vi "Set Tree Items.vi"(8 "error in (no error)":errorcluster, 11 "File Explorer in":refnum<class "File Explorer.lvclass">) -> (0 "error out":errorcluster, 3 "File Explorer out":refnum<class "File Explorer.lvclass">)   [LabVIEW 2019, in "File Explorer.lvlib" / "File Explorer.lvclass"]
uses:
  <vilib>/gpm_packages/@cs/file-explorer-extension/Source/File Explorer/File Explorer/File Explorer.lvclass
  <vilib>/gpm_packages/@cs/file-explorer-extension/Source/File Explorer/File Explorer/File Explorer.lvclass/File Explorer.ctl
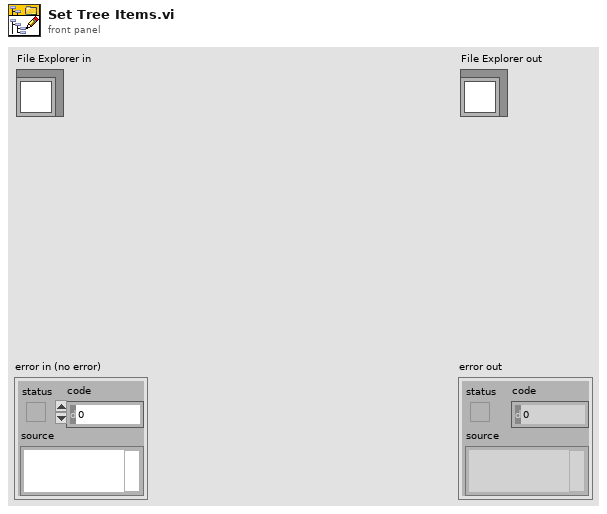
[diagram p1: front panel]
types:
  T1 = cluster{"Left Cell String":string, "Child Text":string[], "Child Tag":string, "Item Indent":i32, "Child Only?":bool, "Glyph Index":i32}[]
  T2 = cluster{"Left Cell String":string, "Child Text":string[], "Child Tag":string, "Item Indent":i32, "Child Only?":bool, "Glyph Index":i32}
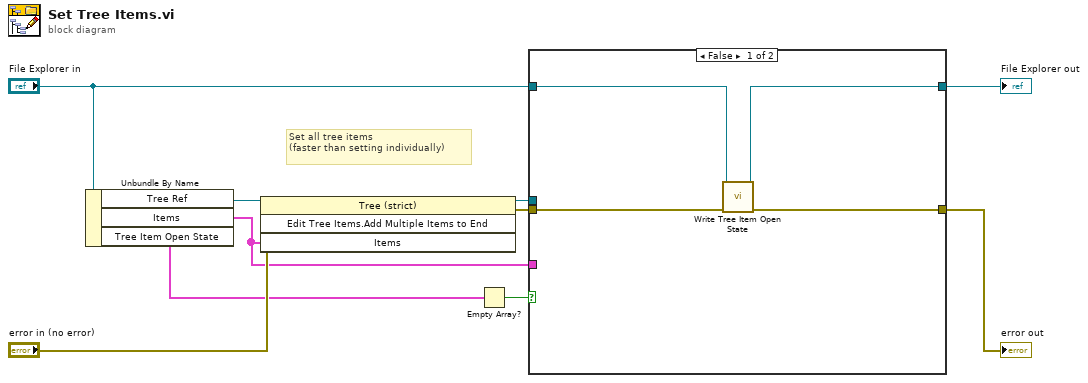
[diagram p0: block diagram]
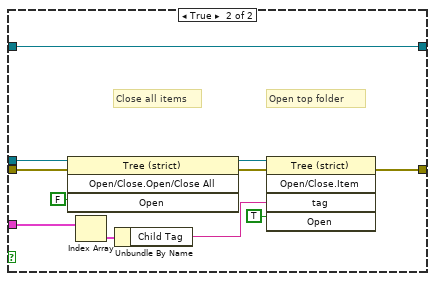
[diagram p2: hidden frame]
diagram:
  # "Set all tree items\n(faster than setting individually)"
  n1 = Unbundle By Name("File Explorer in") -> ("Tree Ref"=w6:refnum<vi>, "Items"=w5:T1, "Tree Item Open State"=w4:cluster{"Tag":string, "Open?":bool}[])
  n2 = invoke class="Tree (strict)" method="Edit Tree Items.Add Multiple Items to End"(reference=w6, error in="error in (no error)", "Items"=w5) -> (reference out=w9:refnum<vi>, error out=w10:errorcluster)  [unwired: 1 in, 2 out]
  n3 = Empty Array?(array=w4) -> (empty?=w3:bool)
  n4 = case shown="False" w3 {
    tunnel: w10 -> [w14 w25]
    tunnel: w9 -> [_ w24]
    tunnel: [w13 w17] -> w7
    tunnel: w5 -> [_ w16]
    tunnel: [w11 w15] -> w1
    tunnel: "File Explorer in" -> [w12 w15]
    frame False {
      n5 = call <vilib>:"Write Tree Item Open State.vi"("error in (no error)"=w14, "File Explorer in"=w12) -> ("error out"=w13:errorcluster, "File Explorer out"=w11:refnum<class "File Explorer.lvclass">)  [unwired: 8 in]
    }
    frame True {
      # "Open top folder"
      # "Close all items"
      n6 = invoke class="Tree (strict)" method="Open/Close.Open/Close All"(reference=w24, error in=w25, "Open"=FALSE ("Open?")) -> (reference out=w22:refnum<vi>, error out=w21:errorcluster)  [unwired: 1 in, 2 out]
      n7 = Index Array(array=w16) -> (element=w20:T2)  [unwired: 1 in]
      n8 = Unbundle By Name(w20) -> ("Child Tag"=w19:string)
      n9 = invoke class="Tree (strict)" method="Open/Close.Item"(reference=w22, error in=w21, "tag"=w19, "Open"=TRUE ("Open?")) -> (error out=w17:errorcluster)  [unwired: 1 in, 4 out]
    }
  }
  "error out" <- w7
  "File Explorer out" <- w1
